vi "Keyence.Cmd.ParametersBank.Get.vi"(6 "Timeout [ms] (1000)":i32=1000, 7 "Bank":u8, 8 "error in":errorcluster, 10 "Cmd":T1, 11 "cID in":refnum<k5>) -> (0 "error out":errorcluster, 1 "OK?":bool, 2 "Response":string, 3 "cID out":refnum<k5>)   [LabVIEW 2016]
uses:
  Keyence.Cmd.ParametersBank.ctl
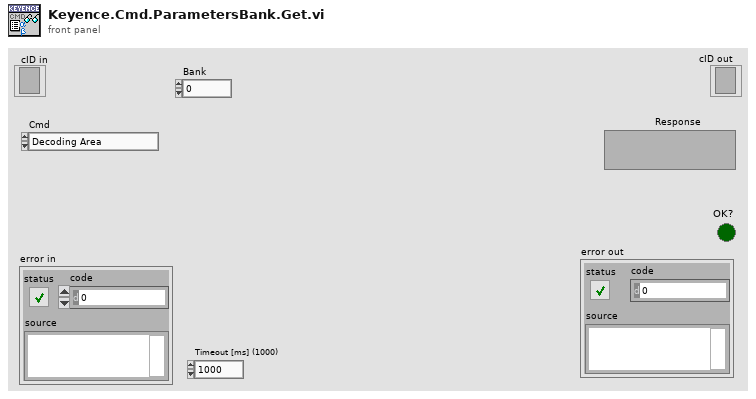
[diagram p1: front panel]
types:
  T1 = typedef "Keyence.Cmd.ParametersBank.ctl" = enum16{"Decoding Area", "Scan.DynamicRange"}
  T2 = enum16{"Standard", "Buffered", "CRLF", "Immediate"}
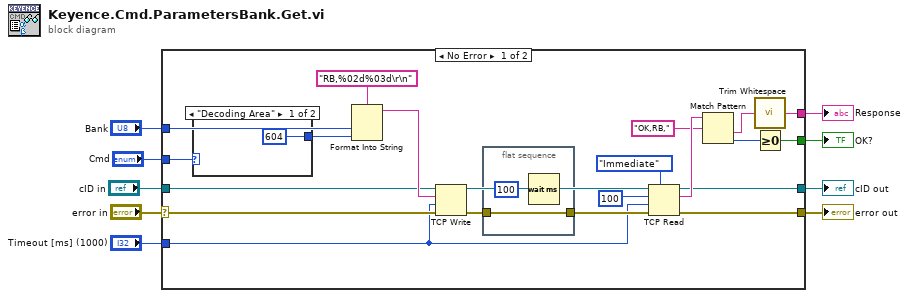
[diagram p0: block diagram]
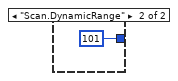
[diagram p2: hidden frame]
diagram:
  n1 = case shown="No Error" "error in" {
    selector: "error in" -> [w13 w35]
    tunnel: "Timeout [ms] (1000)" -> [w11 _]
    tunnel: "Cmd" -> [w30 _]
    tunnel: "Bank" -> [w29 _]
    tunnel: "cID in" -> [w12 w36]
    tunnel: [w23 w36] -> w5
    tunnel: [w24 w35] -> w2
    tunnel: [w14 _] -> w4
    tunnel: [w22 _] -> w3
    frame No Error {
      n2 = case shown="\"Decoding Area\"" w30 {
        tunnel: [604 101] -> w28
        frame "Decoding Area" {
        }
        frame "Scan.DynamicRange" {
        }
      }
      n3 = Format Into String(format string="RB,%02d%03d\r\n", w29, w28) -> (resulting string=w26:string)  [unwired: 2 in, 1 out]
      n4 = TCP Write(connection ID=w12, data in=w26, error in (no error)=w13, 9:w11) -> (connection ID out=w16:refnum<k5>, error out=w18:errorcluster)  [unwired: 1 out]
      n5 = flat-sequence {
        tunnel: w18 -> [w32]
        tunnel: [w32] -> w17
        frame #0 {
          n6 = Wait (ms)(milliseconds to wait=u32 100) -> ()  [unwired: 1 out]
        }
      }
      n7 = TCP Read(connection ID=w16, bytes to read=100, error in (no error)=w17, 7:T2."Immediate" ("mode (standard)"), 9:w11) -> (connection ID out=w23:refnum<k5>, data out=w25:string, error out=w24:errorcluster)
      n8 = Match Pattern(string=w25, regular expression="OK,RB,") -> (after substring=w15:string, offset past match=w21:i32)  [unwired: 1 in, 2 out]
      n9 = call <vilib>:"Trim Whitespace.vi"("string"=w15) -> ("trimmed string"=w14:string)  [unwired: 1 in]
      n10 = Greater Or Equal To 0?(x=w21) -> (x >= 0?=w22:bool)
    }
    frame Error {
    }
  }
  "cID out" <- w5
  "Response" <- w4
  "OK?" <- w3
  "error out" <- w2
